vi "FFT.vi"() -> ()   [LabVIEW 2020]
uses:
  <vilib>/rvi/Analysis/measure/FFT/simModelSupport/niFPGA FFT Outside SCTL Sim Properties.ctl
  <vilib>/rvi/Analysis/measure/FFT/simModelSupport/niFPGA FFT Sim Types.ctl
  <vilib>/rvi/Analysis/measure/FFT/simModelSupport/niFpgaFFTSimArithmeticProperties.ctl
  <vilib>/rvi/Analysis/measure/FFT/simModelSupport/niFpgaFFTSimDfxp.ctl
  <vilib>/fxp/LVFixedPointQuantizationPolicyTypeDef.ctl
  <vilib>/rvi/FXPMathLib/FxpSinAndCos/subVIs/nifxpmath_SinAndCos_SimConfig.ctl
  <vilib>/rvi/DataTransferAndStorage/Container/Common/niFpgaContainerGetUniqueNameForEmu.vi
  <vilib>/rvi/DataTransferAndStorage/Container/Common/niFpgaContainerSetEmuInfo.vi
  <vilib>/rvi/eio/common/nirviEmuReportErrorAndStop.vi
  <vilib>/rvi/interface/RandomDataEmulation/niFpgaRandomDataHandleErrors.vi
  <vilib>/rvi/DataTransferAndStorage/Container/Common/niFpgaContainerExecOnDevCompGetState.vi
  <vilib>/rvi/Emulation/niFpgaEmulationIsFPGAContextNoSignature.vi
  <vilib>/rvi/Emulation/niFpgaSctlEmulationGetInTimedLoop.vi
  <vilib>/rvi/errors/niFpgaSetErrorForExecOnDevCompSimple.vi
  <vilib>/rvi/FIFO/Fifo_Resource/nirvififoEmulationSetSize.vi
  <vilib>/rvi/FIFO/Fifo_Resource/nirviFifoEmulationQueueMgr.vi
  <instcachedir>/0/nirviFifoEmulationQueueMgr_E5CAEC123FF24DC58D834DCA3CDAA9B5.lvgen/nirviFifoEmulationQueueMgr_E5CAEC123FF24DC58D834DCA3CDAA9B5_008.vi
  <vilib>/rvi/FIFO/Fifo_Resource/nirvififoEmulationDetermineInputValidOut.vi
  <vilib>/rvi/FIFO/Fifo_Resource/nirvififoEmulationCreateLock.vi
  <vilib>/rvi/Emulation/niFpgaProcessEmulError.vi
  <vilib>/rvi/FIFO/Fifo_Resource/nirvififoEmulationObtainLock.vi
  <vilib>/rvi/FIFO/Fifo_Resource/nirvififoEmulationReleaseLock.vi
  <vilib>/rvi/occurrence/nirviWaitOnOccurrenceBase.vi
  <vilib>/rvi/errors/nirviReportUnexpectedCaseInternalError.vi
  <vilib>/rvi/errors/nirviReportUnexpectedCaseInternalError (U32).vi
  <vilib>/Utility/error.llb/Clear Errors.vi
  <vilib>/rvi/Emulation/niFpgaGetClockAttributes.vi
  <vilib>/rvi/Emulation/niFpgaEmulationReportErrorSimple.vi
  <vilib>/rvi/Analysis/measure/FFT/simModelSupport/niFpgaFFTSimModelOutsideSCTLCore.vi
  <vilib>/rvi/FXPMathLib/FxpSinAndCos/simVIs/DllFxpSinAndCosTemp_sub.vi
  <vilib>/rvi/Emulation/niFpgaCriticalErrorInLSC.vi
  <vilib>/rvi/LocalResourceManager/LocalResourceManager.xnode
  <vilib>/rvi/DataTransferAndStorage/Container/XNode/niFpgaContainer.xnode
  <vilib>/rvi/interface/RandomDataEmulation/nirviRandomDataFpgaReadWriteTemplate.vi
  <vilib>/rvi/FIFO/Fifo_Resource/niFpgaFifoEmulationRefIn.vi
  <vilib>/rvi/Analysis/measure/FFT/XNode/niFpgaFFT.xnode
  <vilib>/rvi/FXPMathLib/FxpSinAndCos/XNode/nifxpmath_SinAndCos.xnode
panel:
  out "Numeric":i32
  out "appended array":fxp<+/-,24,7>[](array[numeric])
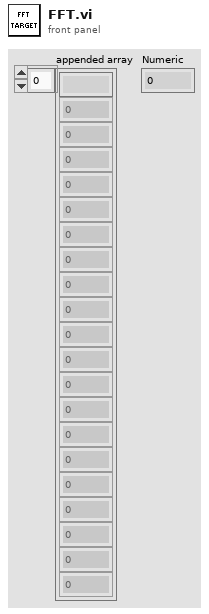
[diagram p1: front panel]
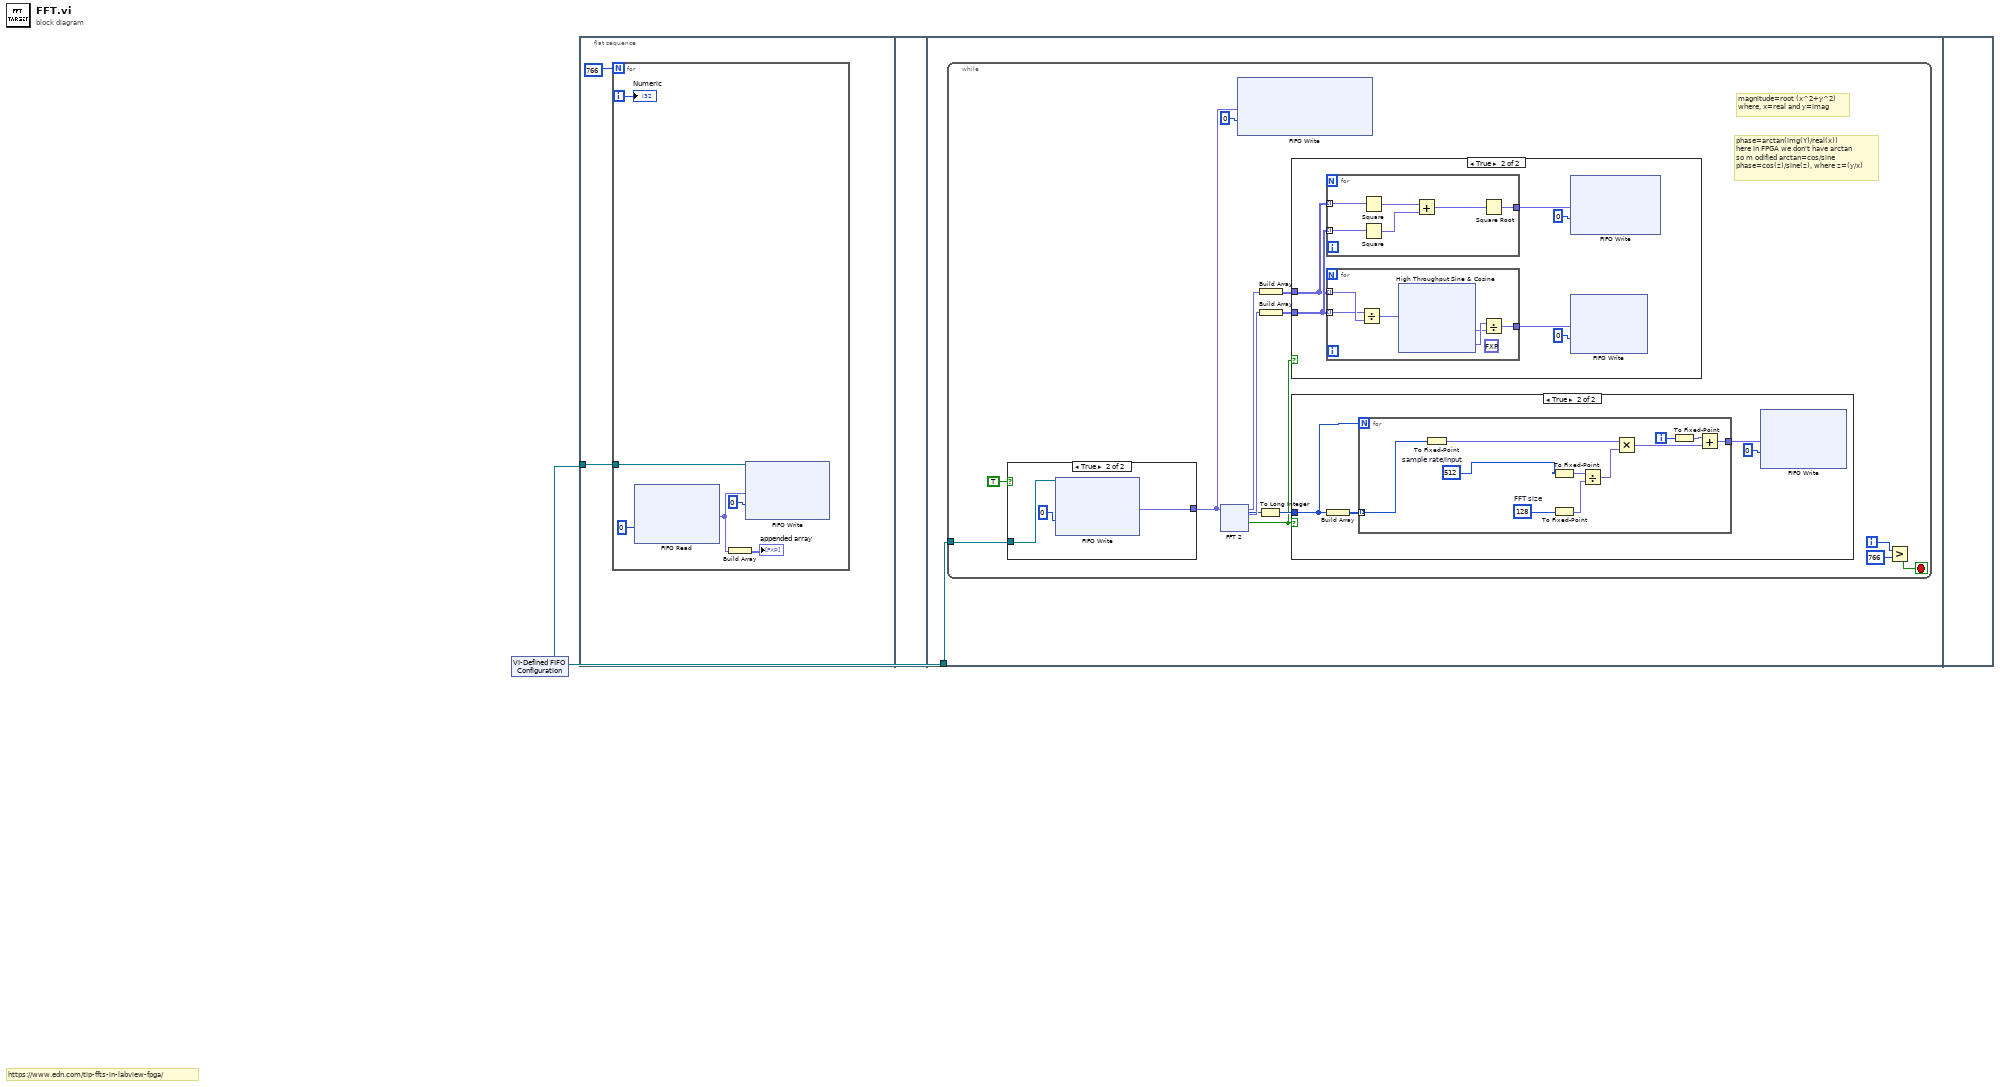
[diagram p0: block diagram]
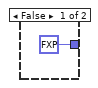
[diagram p4: hidden frame]
diagram:
  # "https://www.edn.com/tip-ffts-in-labview-fpga/"
  n1 = xnode "VI-Defined FIFO Configuration"() -> ("FIFO Out"=w1:refnum<k21>)
  n2 = flat-sequence {
    tunnel: w1 -> [w3]
    tunnel: w1 -> [w10]
    frame #0 {
      n3 = for {
        N: 766 -> [_]
        tunnel: w3 -> [w8]
        i -> [w4]
        n4 = xnode ("FIFO Read")("Timeout"=0) -> ("Element"=w6:fxp<+/-,24,7>)  [unwired: 1 in, 2 out]
        n5 = Build Array(w6) -> (→"appended array":fxp<+/-,24,7>[])
        n6 = xnode ("FIFO Write")("Element"=w6, "Timeout"=0, "FIFO In"=w8) -> ()  [unwired: 2 out]
        "Numeric" <- w4
      }
    }
    frame #1 {
    }
    frame #2 {
      n7 = while {
        tunnel: w10 -> [w22]
        i -> [w15]
        stop <- w23 stop-if-true
        # "magnitude=root (x^2+y^2)\nwhere, x=real and y=imag"
        # "phase=arctan(img(Y)/real(x))\nhere in FPGA we don't have arctan\nso m odified arctan=cos/sine\nphase=cos(z)/sine(z), where z=(y/x)"
        n8 = case shown="True" TRUE {
          tunnel: w22 -> [_ w91]
          tunnel: [fxp<+/-,24,7> 0.0 ("Element") w89] -> w17
          frame False {
          }
          frame True {
            n9 = xnode ("FIFO Write")("Timeout"=0, "FIFO In"=w91) -> ("Element"=w89:fxp<+/-,24,7>)  [unwired: 2 out]
          }
        }
        n10 = xnode ("FFT 2")("real data in"=w17) -> ("data index"=w12:u16, "real data out"=w16:fxp<+/-,32,15>, "imaginary data out"=w14:fxp<+/-,32,15>, "output valid"=w11:bool)  [unwired: 2 in]
        n11 = xnode ("FIFO Write")("Element"=w17, "Timeout"=0) -> ()  [unwired: 1 in, 2 out]
        n12 = To Long Integer(number=w12) -> (32bit integer=w13:i32)
        n13 = Build Array(w16) -> (w19:fxp<+/-,32,15>[])
        n14 = Build Array(w14) -> (w20:fxp<+/-,32,15>[])
        n15 = case shown="True" w11 {
          tunnel: w20 -> [_ w41]
          tunnel: w19 -> [_ w40]
          frame False {
          }
          frame True {
            n16 = for {
              tunnel: w40 -> [w87] mode=indexing
              tunnel: [w82] -> w42
              tunnel: w41 -> [w83] mode=indexing
              n17 = Square(x=w87) -> (x^2=w86:fxp<+,63,29>)
              n18 = Square(x=w83) -> (x^2=w85:fxp<+,63,29>)
              n19 = Add(x=w86, y=w85) -> (x+y=w84:fxp<+,64,30>)
              n20 = Square Root(x=w84) -> (sqrt(x)=w82:fxp<+/-,32,16>)
            }
            n21 = for {
              tunnel: w40 -> [w47] mode=indexing
              tunnel: w41 -> [w46] mode=indexing
              tunnel: [w49] -> w44
              (unwired) fxp<+/-,32,16> 0.0 ("fixed-point type")
              n22 = Divide(x=w46, y=w47) -> (x/y=w48:fxp<+/-,32,16>)
              n23 = xnode "High Throughput Sine & Cosine"("x (pi)"=w48) -> ("sin(x)"=w50:fxp<+/-,32,2>, "cos(x)"=w51:fxp<+/-,32,2>)
              n24 = Divide(x=w51, y=w50) -> (x/y=w49:fxp<+/-,32,16>)
            }
            n25 = xnode ("FIFO Write")("Element"=w42, "Timeout"=0) -> ()  [unwired: 1 in, 2 out]
            n26 = xnode ("FIFO Write")("Element"=w44, "Timeout"=0) -> ()  [unwired: 1 in, 2 out]
          }
        }
        n27 = case shown="True" w11 {
          tunnel: w13 -> [_ w28]
          frame False {
          }
          frame True {
            n28 = Build Array(w28) -> (w27:i32[])
            n29 = for {
              N: w28 -> [_]
              tunnel: w27 -> [w33] mode=indexing
              tunnel: [w37] -> w26
              i -> [w31]
              w29 = 512  # sample rate/input
              w35 = 128  # FFT size
              n30 = To Fixed-Point(number=w33) -> (fixed-point=w32:fxp<+/-,32,32>)  [unwired: 1 in]
              n31 = To Fixed-Point(number=w29) -> (fixed-point=w36:fxp<+/-,32,32>)  [unwired: 1 in]
              n32 = To Fixed-Point(number=w35) -> (fixed-point=w34:fxp<+/-,32,32>)  [unwired: 1 in]
              n33 = Divide(x=w36, y=w34) -> (x/y=w39:fxp<+/-,32,16>)
              n34 = Multiply(x=w32, y=w39) -> (x*y=w38:fxp<+/-,64,48>)
              n35 = To Fixed-Point(number=w31) -> (fixed-point=w30:fxp<+/-,32,32>)  [unwired: 1 in]
              n36 = Add(x=w30, y=w38) -> (x+y=w37:fxp<+/-,32,16>)
            }
            n37 = xnode ("FIFO Write")("Element"=w26, "Timeout"=0) -> ()  [unwired: 1 in, 2 out]
          }
        }
        n38 = Greater?(x=w15, y=766 ("Timeout")) -> (0:w23:bool)
      }
    }
    frame #3 {
    }
  }
